vi "Follow Wall.vi"(8 "Course Stage":i32=3, 11 "Event":T1=enum."Start Button Pressed") -> (3 "Next State":u16=6)   [LabVIEW 2017]
uses:
  Event.ctl
  State.ctl
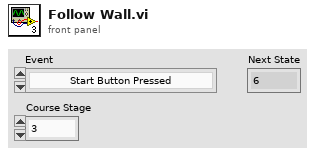
[diagram p1: front panel]
types:
  T1 = typedef "Event.ctl" = enum16{"None", "Zig Zag Finished", "Start Obstacle Avoidance", "Start Button Pressed", "Black & Yellow Tape Touched", "Black & Yellow Tape Passed", "Green Tape Crossed", "Red Tape Touched", "Rough Terrain Touched", "Black Tape Crossed", "Tape Edge Too Close", "Wall Too Close", "Rough Terrain Passed", "Ramp Passed", "Stop Button Pressed", "Recentered", "End Zone Wait Timed Out"}
  T2 = typedef "State.ctl" = enum16{"Wait", "Recenter", "Follow Wall", "Zig Zag", "Ramp", "Cross Rough Terrain", "Stagger Stop", "Obstacle Avoidance"}
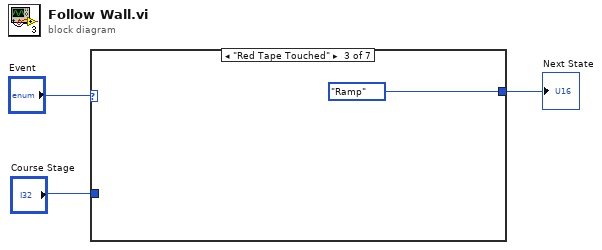
[diagram p0: block diagram]
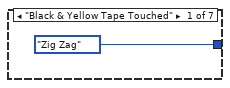
[diagram p2: hidden frame]
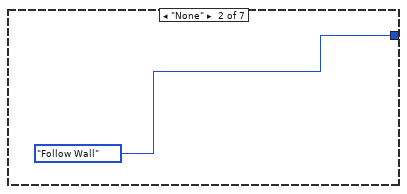
[diagram p3: hidden frame]
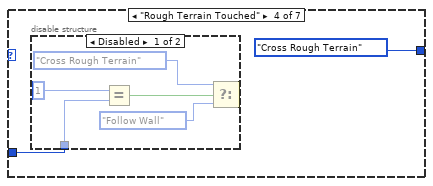
[diagram p4: hidden frame]
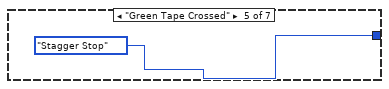
[diagram p6: hidden frame]
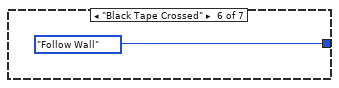
[diagram p7: hidden frame]
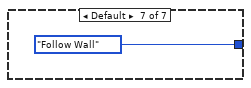
[diagram p8: hidden frame]
diagram:
  n1 = case shown="\"Red Tape Touched\"" "Event" {
    tunnel: [State."Zig Zag" ("State") State."Follow Wall" ("State") State."Ramp" ("State") State."Cross Rough Terrain" ("State") State."Stagger Stop" ("t") State."Follow Wall" ("State") State."Follow Wall" ("State")] -> w2
    tunnel: "Course Stage" -> [_ _ _ w8 _ _ _]
    frame "Black & Yellow Tape Touched" {
    }
    frame "None" {
    }
    frame "Red Tape Touched" {
    }
    frame "Rough Terrain Touched" {
      n2 = disable-structure shown="Disabled" {
        disable-tunnel: w8 -> [w9 _]
        frame Disabled {
          n3 = Equal?(x=1, y=w9) -> (x = y?=w12:bool)
          n4 = Select(t=State."Cross Rough Terrain", s=w12, f=State."Follow Wall" ("State")) -> ()  [unwired: 1 out]
        }
        frame Enabled {
        }
      }
    }
    frame "Green Tape Crossed" {
    }
    frame "Black Tape Crossed" {
    }
    frame Default {
    }
  }
  "Next State" <- w2
